vi "Enumerate Format Names.vi"(8 "error in (no error)":errorcluster, 11 "CameraManager":refnum<data-value>) -> (0 "error out":errorcluster, 2 "Formats":map{u32, string}(c390), 3 "CameraManager (duplicate)":refnum<data-value>)   [LabVIEW 2020, in "g_ar_toolkit.capture.lvlib" / "CameraManager.lvclass"]
uses:
  CameraManager.lvclass
  CameraManager.lvclass/CameraManager.ctl
  <vilib>/Utility/error.llb/Error Cluster From Error Code.vi
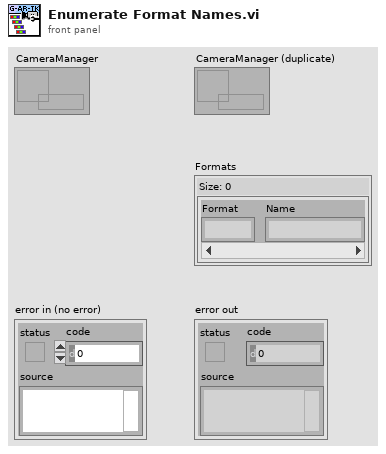
[diagram p1: front panel]
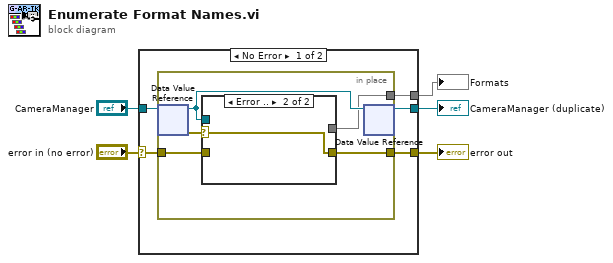
[diagram p0: block diagram]
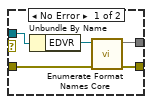
[diagram p2: hidden frame]
diagram:
  n1 = case shown="No Error" "error in (no error)" {
    selector: "error in (no error)" -> [w6 w23]
    tunnel: [w9 w23] -> w4
    tunnel: [w8 w22] -> w2
    tunnel: "CameraManager" -> [w10 w22]
    tunnel: [w7 _] -> w1
    frame No Error {
      n2 = in-place {
        in-place-border: [w14] -> w9
        in-place-border: [w12] -> w7
        in-place-border: w6 -> [w11]
        n3 = in-place-dvr #1(w10) -> (w13:refnum<class "CameraManager.lvclass">, w15:errorcluster)
        n4 = case shown="Error .." w15 {
          selector: w15 -> [_ w21]
          tunnel: [w19 w21] -> w14
          tunnel: w13 -> [w18 _]
          tunnel: [w17 _] -> w12
          tunnel: w11 -> [w16 _]
          frame No Error {
            n5 = Unbundle By Name(w18) -> ("EDVR"=w20:refnum<data-value>)
            n6 = call "Enumerate Format Names Core.vi"("error in (no error)"=w16, "Data Value Reference in"=w20) -> ("error out"=w19:errorcluster, "Map"=w17:map{u32, string})  [unwired: 8 in]
          }
          frame Error {
          }
        }
        n7 = in-place-dvr #1(w13) -> (w8:refnum<data-value>)  [unwired: 1 out]
      }
    }
    frame Error {
    }
  }
  "error out" <- w4
  "CameraManager (duplicate)" <- w2
  "Formats" <- w1
